vi "Apply Ethernet Configuration.vi"(7 "Restart (T)":bool=TRUE, 8 "error in (no error)":errorcluster, 10 "Ethernet Settings":T1={"IP Address"="192.168.1.100", "TCP (Command) Port"=12345, "TCP (Command) Read Interval (ms)"=10, "UDP (Reporting) Port"=54321, "UDP (Reporting) Write Interval (ms)"=5, "UDP Data Broadcast Enable"=FALSE}, 11 "Ethernet in":refnum<class "ENET_BS1201.lvclass">) -> (0 "error out":errorcluster, 3 "Ethernet out":refnum<class "ENET_BS1201.lvclass">)   [LabVIEW 2021, in "BS120x Driver.lvlib" / "ENET_BS1201.lvclass"]
doc: "Sends the configuration updates to the Battery Simulator 1200, and automatically triggers a restart.\nFor BS1201: the Restart input is no longer required. Restart is automatic on the BS1201 when configuration changes are made.\n(c) 2019 Bloomy Controls, Inc. All rights reserved."
uses:
  ENET_BS1201.lvclass
  TypeDefs/Ethernet Settings.ctl
  ENET_BS1201.lvclass/ENET_BS1201.ctl
  BS120x.lvclass
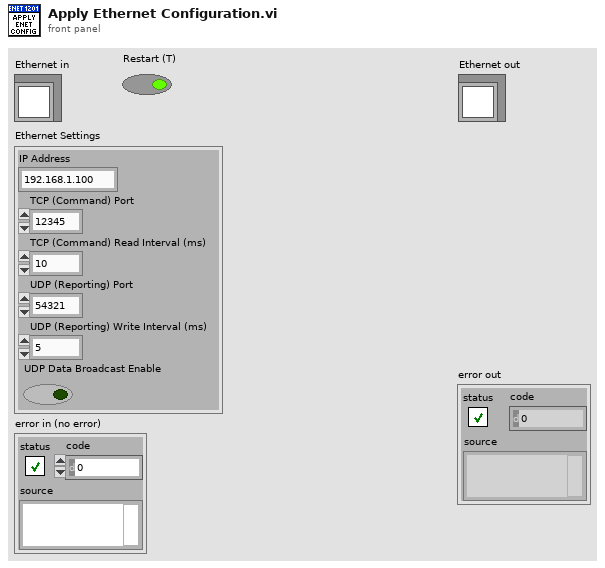
[diagram p1: front panel]
types:
  T1 = typedef "BS120x Driver.lvlib/BS120x.lvclass/Ethernet Settings.ctl" = cluster{"IP Address":string, "TCP (Command) Port":u16, "TCP (Command) Read Interval (ms)":u32, "UDP (Reporting) Port":u16, "UDP (Reporting) Write Interval (ms)":u32, "UDP Data Broadcast Enable":bool}
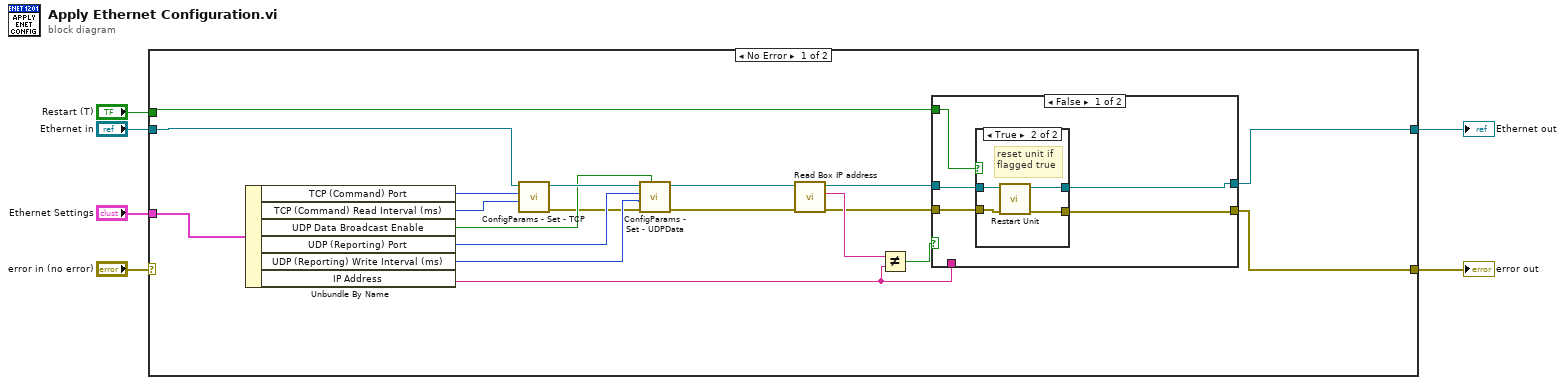
[diagram p0: block diagram]
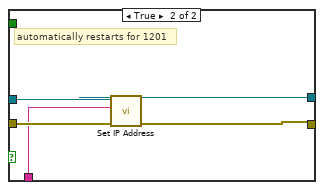
[diagram p3: hidden frame]
diagram:
  n1 = case shown="No Error" "error in (no error)" {
    selector: "error in (no error)" -> [_ w43]
    tunnel: [w17 w43] -> w5
    tunnel: [w16 w42] -> w3
    tunnel: "Ethernet in" -> [w24 w42]
    tunnel: "Ethernet Settings" -> [w25 _]
    tunnel: "Restart (T)" -> [w13 _]
    frame No Error {
      n2 = Unbundle By Name(w25) -> ("TCP (Command) Port"=w23:u16, "TCP (Command) Read Interval (ms)"=w22:u32, "UDP Data Broadcast Enable"=w19:bool, "UDP (Reporting) Port"=w20:u16, "UDP (Reporting) Write Interval (ms)"=w18:u32, "IP Address"=w15:string)
      n3 = call-dynamic "ConfigParams - Set - TCP.vi"("TCPLoopTime_mS"=w22, "TCPCommandPort"=w23, "Ethernet in"=w24) -> ("error out"=w9:errorcluster, "Ethernet out"=w21:refnum<class "ENET_BS1201.lvclass">)  [unwired: 7 in]
      n4 = call-dynamic "ConfigParams - Set - UDPData.vi"("UDP Data Enable"=w19, "error in (no error)"=w9, "UDPDataPeriod_mS"=w18, "UDP Data Port"=w20, "Ethernet in"=w21) -> ("error out"=w7:errorcluster, "Ethernet out"=w8:refnum<class "ENET_BS1201.lvclass">)  [unwired: 5 in]
      n5 = call-dynamic "Read Box IP address.vi"("error in (no error)"=w7, "ENET_BS120x in"=w8) -> ("error out"=w10:errorcluster, "Box IP address"=w12:string, "ENET_BS120x out"=w11:refnum<class "ENET_BS1201.lvclass">)  [unwired: 7 in]
      n6 = Not Equal?(x=w12, y=w15) -> (x != y?=w14:bool)
      n7 = case shown="False" w14 {
        tunnel: w10 -> [w30 w41]
        tunnel: w11 -> [w29 w40]
        tunnel: w15 -> [_ w39]
        tunnel: [w27 w37] -> w17
        tunnel: [w28 w38] -> w16
        tunnel: w13 -> [w26 _]
        frame False {
          n8 = case shown="True" w26 {
            tunnel: w30 -> [w31 w34]
            tunnel: w29 -> [w32 w36]
            tunnel: [w32 w35] -> w28
            tunnel: [w31 w33] -> w27
            frame False {
            }
            frame True {
              # "reset unit if\nflagged true"
              n9 = call-dynamic "Restart Unit.vi"("error in (no error)"=w34, "ENET in"=w36) -> ("error out"=w33:errorcluster, "ENET out"=w35:refnum<class "ENET_BS1201.lvclass">)  [unwired: 8 in]
            }
          }
        }
        frame True {
          # "automatically restarts for 1201"
          n10 = call-dynamic "Set IP Address.vi"("error in (no error)"=w41, "IP Address"=w39, "ENET in"=w40) -> ("error out"=w37:errorcluster, "ENET out"=w38:refnum<class "ENET_BS1201.lvclass">)  [unwired: 7 in]
        }
      }
    }
    frame Error {
    }
  }
  "error out" <- w5
  "Ethernet out" <- w3
